vi "ELVIS III v1.0 Write Read SPI.vi"(8 "error in (no error)":errorcluster, 9 "Data In":u16[](array[numeric]), 10 "Channel":T1, 11 "myRIO Ref In":T2) -> (0 "error out":errorcluster, 1 "Data Out":u16[](array[numeric]), 3 "myRIO Ref Out":T2)   [LabVIEW 2021]
uses:
  <vilib>/myRIO/Common/Instrument Driver Framework/Utilities/typedefs/myRIO v1.0 Reference.ctl
  <vilib>/myRIO/Common/Instrument Driver Framework/Utilities/typedefs/Generic FPGA Reference.ctl
  <vilib>/myRIO/Common/Instrument Driver Framework/myRIO v1.0/SPI/typedefs/SPI Channels Enum.ctl
  <vilib>/myRIO/Common/Instrument Driver Framework/myRIO v1.0/SPI/typedefs/SPI Channels FPGA Reference.ctl
  <vilib>/rvi/errors/niLvFpgaAdjustHostInterfaceError.vi
  <vilib>/RVI Host/nirviSupport.llb/nirviErrorClusterFromErrorCode.vi
  <vilib>/rvi/interface/nirviReadWriteControl/nirviReadWriteControl.xnode
  <vilib>/rvi/interface/nirviMethod/nirviMethod.xnode
  <vilib>/rvi/interface/Simulation/niFpgaSimulationCallBeginRW.vi
  NiFpgaLv.dll
  <vilib>/rvi/interface/nirviMethod/StockFPGA_InlinedMethodWaitForSingleIRQ.vi
  <vilib>/FPGAPlugInAG/Dynamic/niLvFpga_WaitOnIrq_Dynamic.vi
  <vilib>/FPGAPlugInAG/Dynamic/niLvFpga_AcknowledgeIrq_Dynamic.vi
panel:
  # "This VI writes an array of data to the SPI Data Out register (SPIn.SPDO) and reads an array of data from the SPI Data In register (SPIn.SPDI) for a particular SPI channel (n). The data is written/read one value at a time. Please see Block Diagram for details."
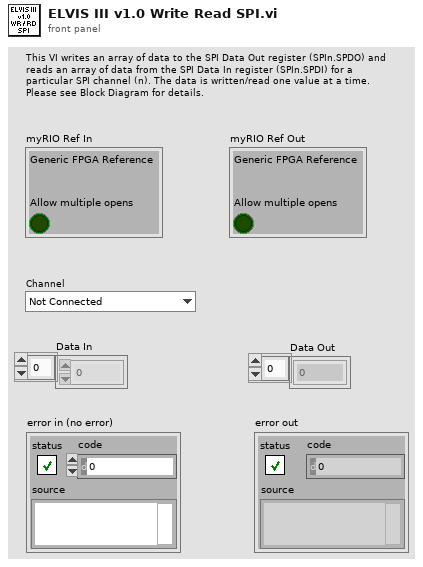
[diagram p1: front panel]
types:
  T1 = typedef "SPI Channels Enum.ctl" = enum16{"Not Connected", "A/SPI", "B/SPI", "SPI/SPI"}
  T2 = typedef "myRIO v1.0 Reference.ctl" = cluster{"Generic FPGA Reference":T3, "Allow multiple opens":bool}
  T3 = typedef "Generic FPGA Reference.ctl" = refnum<k20>
  T4 = typedef "SPI Channels FPGA Reference.ctl" = refnum<k20>
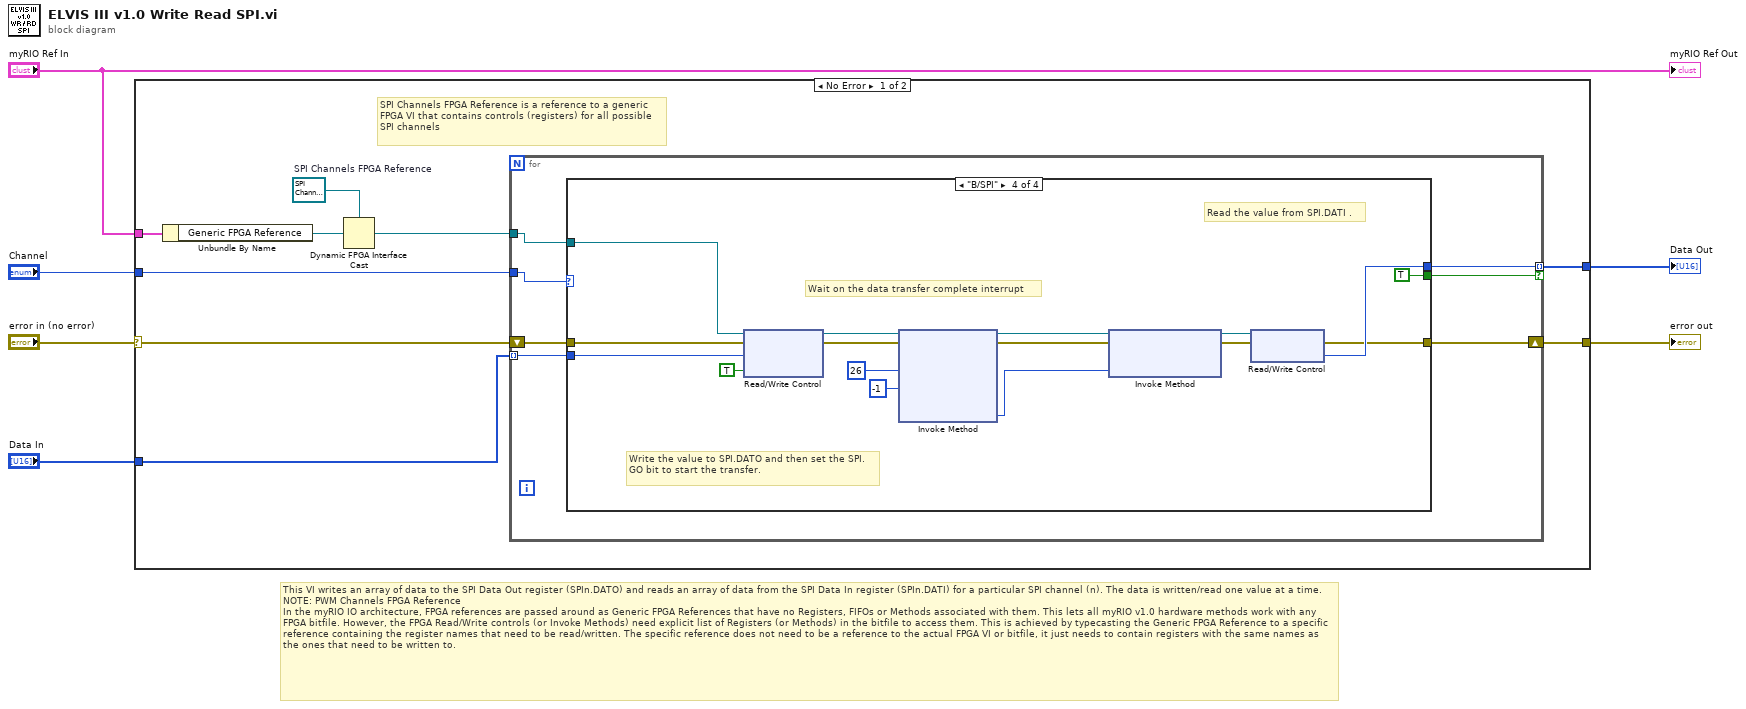
[diagram p0: block diagram]
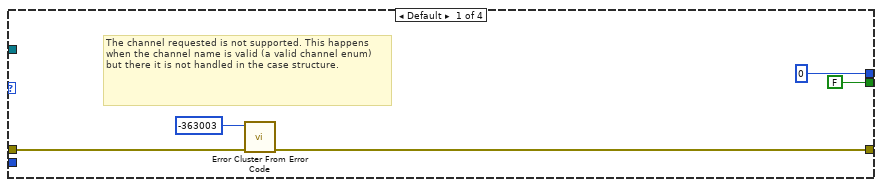
[diagram p2: hidden frame]
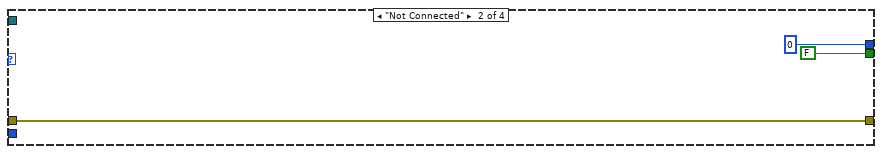
[diagram p3: hidden frame]
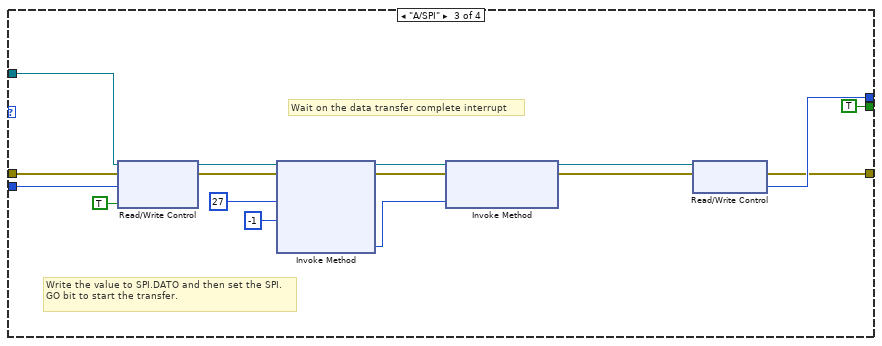
[diagram p4: hidden frame]
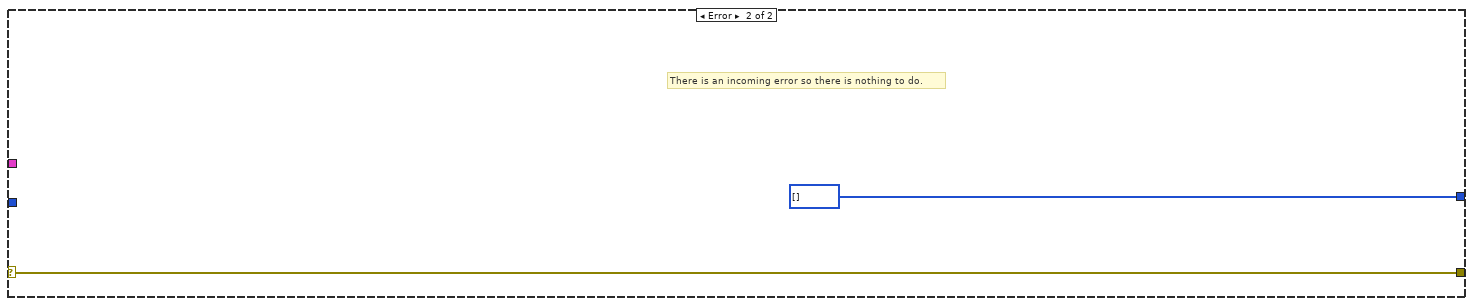
[diagram p5: hidden frame]
diagram:
  # "This VI writes an array of data to the SPI Data Out register (SPIn.DATO) and reads an array of data from the SPI Data In register (SPIn.DATI) for a particular SPI channel (n). The data is written/read one value at a time.\nNOTE: PWM Channels FPGA Reference\nIn the myRIO IO architecture, FPGA references are passed around as Generic FPGA References that have no Registers, FIFOs or Methods associated with them. This lets all myRIO v1.0 hardware methods work with any FPGA bitfile. However, the FPGA Read/Write controls (or Invoke Methods) need explicit list of Registers (or Methods) in the bitfile to access them. This is achieved by typecasting the Generic FPGA Reference to a specific reference containing the register names that need to be read/written. The specific reference does not need to be a reference to the actual FPGA VI or bitfile, it just needs to contain registers with the same names as the ones that need to be written to."
  n1 = case shown="No Error" "error in (no error)" {
    selector: "error in (no error)" -> [w8 w64]
    tunnel: [w12 u16[] [] ("t")] -> w6
    tunnel: "Channel" -> [w14 _]
    tunnel: [w13 w64] -> w4
    tunnel: "Data In" -> [w11 _]
    tunnel: "myRIO Ref In" -> [w10 _]
    frame No Error {
      w15 = T4 refnum  # SPI Channels FPGA Reference
      # "SPI Channels FPGA Reference is a reference to a generic FPGA VI that contains controls (registers) for all possible SPI channels"
      n2 = Unbundle By Name(w10) -> ("Generic FPGA Reference"=w9:T3)
      n3 = Dynamic FPGA Interface Cast(Session In=w15, Type=w9) -> (Session Out=w7:T4)
      n4 = for {
        tunnel: w7 -> [w22]
        tunnel: w14 -> [w19]
        tunnel: w11 -> [w18] mode=indexing
        tunnel: [w17] -> w12 mode=indexing if=w16
        shift-right: [w20] -> w13
        shift-left: w8 -> [w21]
        n5 = case shown="\"B/SPI\"" w19 {
          tunnel: w21 -> [w25 w30 w43 w61]
          tunnel: [w26 w30 w38 w55] -> w20
          tunnel: w22 -> [_ _ w44 w62]
          tunnel: w18 -> [_ _ w42 w60]
          tunnel: [u16 0 ("SPI1.SPDI") u16 0 ("SPI1.SPDI") w40 w57] -> w17
          tunnel: [FALSE FALSE TRUE TRUE] -> w16
          frame Default {
            # "The channel requested is not supported. This happens when the channel name is valid (a valid channel enum) but there it is not handled in the case structure."
            n6 = call <vilib>:"Error Cluster From Error Code.vi"("error in (no error)"=w25, "error code (0)"=-363003) -> ("error out"=w26:errorcluster)  [unwired: 7 in]
          }
          frame "Not Connected" {
          }
          frame "A/SPI" {
            # "Wait on the data transfer complete interrupt"
            # "Write the value to SPI.DATO and then set the SPI.GO bit to start the transfer."
            n7 = xnode "Read/Write Control"("FPGA VI Reference In"=w44, "error in"=w43, "SPI.A.DATO"=w42, "SPI.A.GO"=TRUE) -> ("FPGA VI Reference Out"=w46:T4, "error out"=w45:errorcluster)
            n8 = xnode "Invoke Method"("FPGA VI Reference In"=w46, "error in"=w45, "IRQ Number(s)"=27, "Timeout (ms)"=-1) -> ("FPGA VI Reference Out"=w35:T4, "error out"=w32:errorcluster, "IRQ(s) Asserted"=w33:i32)  [unwired: 1 out]
            n9 = xnode "Invoke Method"("FPGA VI Reference In"=w35, "error in"=w32, "IRQ Number(s)"=w33) -> ("FPGA VI Reference Out"=w36:T4, "error out"=w41:errorcluster)
            n10 = xnode "Read/Write Control"("FPGA VI Reference In"=w36, "error in"=w41) -> ("error out"=w38:errorcluster, "SPI.A.DATI"=w40:u16)  [unwired: 1 out]
          }
          frame "B/SPI" {
            # "Wait on the data transfer complete interrupt"
            # "Read the value from SPI.DATI ."
            # "Write the value to SPI.DATO and then set the SPI.GO bit to start the transfer."
            n11 = xnode "Read/Write Control"("FPGA VI Reference In"=w62, "error in"=w61, "SPI.B.DATO"=w60, "SPI.B.GO"=TRUE) -> ("FPGA VI Reference Out"=w48:T4, "error out"=w49:errorcluster)
            n12 = xnode "Invoke Method"("FPGA VI Reference In"=w48, "error in"=w49, "IRQ Number(s)"=26, "Timeout (ms)"=-1) -> ("FPGA VI Reference Out"=w53:T4, "error out"=w50:errorcluster, "IRQ(s) Asserted"=w51:i32)  [unwired: 1 out]
            n13 = xnode "Invoke Method"("FPGA VI Reference In"=w53, "error in"=w50, "IRQ Number(s)"=w51) -> ("FPGA VI Reference Out"=w58:T4, "error out"=w59:errorcluster)
            n14 = xnode "Read/Write Control"("FPGA VI Reference In"=w58, "error in"=w59) -> ("error out"=w55:errorcluster, "SPI.B.DATI"=w57:u16)  [unwired: 1 out]
          }
        }
      }
    }
    frame Error {
      # "There is an incoming error so there is nothing to do."
    }
  }
  "error out" <- w4
  "Data Out" <- w6
  "myRIO Ref Out" <- "myRIO Ref In"
